vi "Modules - Station.vi"(8 "error in":errorcluster) -> (0 "error out":errorcluster)   [LabVIEW 2019]
uses:
  Controls/Station - Tab Test Type.ctl
  Controls/Station - Test Type.ctl
  Controls/Station-state.ctl
  Controls/Station - Data Structure.ctl
  Controls/eFGV States.ctl
  <vilib>/Utility/miscctls.llb/LVRowAndColumnTypeDef.ctl
  Controls/Global - Channel.vi
  Controls/Global - Unit.vi
  Controls/Global - Device.vi
  Controls/Global - Rendezvous.vi
panel:
  out "ID":string
  in  "Refresh Button":bool
  out "Main Tab":enum32{"Blank", "Edit"}(tab)
  out "Sub Tab":T1
  out "Unit PPT Triaxial Shear":string caption="Cell Pressure Transducer"
  out "Unit Disp Triaxial Shear":string caption="Cell Pressure Transducer"
  out "Unit LT Triaxial Shear":string caption="Cell Pressure Transducer"
  out "Unit VC Triaxial Shear":string caption="Cell Pressure Transducer"
  out "Unit BPT Triaxial Shear":string caption="Cell Pressure Transducer"
  out "Unit CPT Triaxial Shear":string caption="Cell Pressure Transducer"
  in  "VLC Triaxial Shear":u16(ring) caption="Vertical Load Control" items=["Please Select"]
  in  "BPC Triaxial Shear":u16(ring) caption="Back Pressure Control" items=["Please Select"]
  out "Disp Triaxial Shear":sgl caption="Dispalcement" format="%.5f"
  out "PPT Triaxial Shear":sgl caption="Pore Pressure Transduser" format="%.5f"
  out "LT Triaxial Shear":sgl caption="Load Tranduser" format="%.5f"
  out "BPT Triaxial Shear":sgl caption="Back Pressure Transducer" format="%.5f"
  out "VC Triaxial Shear":sgl caption="Volume Change" format="%.5f"
  out "CPT Triaxial Shear":sgl caption="Cell Pressure Transducer" format="%.5f"
  in  "CPC Triaxial Shear":u16(ring) caption="Cell Pressure Control" items=["Please Select"]
  in  "VLC Triaxial UU":u16(ring) caption="Vertical Load Control" items=["Please Select"]
  out "CPT Triaxial UU":sgl caption="Cell Pressure" format="%.5f"
  out "VLT Triaxial UU":sgl caption="Vertical Load" format="%.5f"
  out "PPT Triaxial UU":sgl caption="Pore Pressure" format="%.5f"
  out "Disp Triaxial UU":sgl caption="Displacement" format="%.5f"
  in  "CPC Triaxial UU":u16(ring) caption="Cell Pressure Control" items=["Please Select"]
  out "Unit CPT Triaxial UU":string caption="Cell Pressure Transducer"
  out "Unit VLT Triaxial UU":string caption="Cell Pressure Transducer"
  out "Unit Disp Triaxial UU":string caption="Cell Pressure Transducer"
  out "Unit PPT Triaxial UU":string caption="Cell Pressure Transducer"
  in  "HLC Shearbox":u16(ring) caption="Horinzontal Load Control" items=["Please Select"]
  out "LT Shearbox":sgl caption="Vertical Load Tranducer" format="%.5f"
  out "Disp Shearbox":sgl caption="Vertical Dispalcement" format="%.5f"
  out "H Dis Shearbox":sgl caption="Horizontal Dispalcement" format="%.5f"
  out "HLT Shearbox":sgl caption="Horinzontal Load Tranducer" format="%.5f"
  in  "VLC Shearbox":u16(ring) caption="Vertical Load Control" items=["Please Select"]
  out "Unit LT Shearbox":string caption="Cell Pressure Transducer"
  out "Unit Disp Shearbox":string caption="Cell Pressure Transducer"
  out "Unit HLT Shearbox":string caption="Cell Pressure Transducer"
  out "Unit H Dis Shearbox":string caption="Cell Pressure Transducer"
  in  "BPC2 Permeability":u16(ring) caption="Back Pressure 2 Control" items=["Please Select"]
  in  "BPC Permeability":u16(ring) caption="Back Pressure Control" items=["Please Select"]
  out "BPT2 Permeability":sgl caption="Back Pressure 2" format="%.5f"
  out "PPT Permeability":sgl caption="Pore Pressure" format="%.5f"
  out "OVC Permeability":sgl caption="Outlet Volume Change" format="%.5f"
  out "BPT Permeability":sgl caption="Back Pressure" format="%.5f"
  out "IVC Permeability":sgl caption="Inlet Volume Change" format="%.5f"
  out "CPT Permeability":sgl caption="Cell Pressure" format="%.5f"
  in  "CPC Permeability":u16(ring) caption="Cell Pressure Control" items=["Please Select"]
  out "Unit CPT Permeability":string caption="Cell Pressure Transducer"
  out "Unit BPT Permeability":string caption="Cell Pressure Transducer"
  out "Unit IVC Permeability":string caption="Cell Pressure Transducer"
  out "Unit BPT2 Permeability":string caption="Cell Pressure Transducer"
  out "Unit OVC Permeability":string caption="Cell Pressure Transducer"
  out "Unit PPT Permeability":string caption="Cell Pressure Transducer"
  out "Disp Consolidation":sgl caption="Dispalcement"
  out "LT Consolidation":sgl caption="Load Tranducer"
  in  "VLC Consolidation":u16(ring) caption="Vertical Load  Control" items=["Please Select"]
  out "Unit LT Consolidation":string caption="Cell Pressure Transducer"
  out "Unit Disp Consolidation":string caption="Cell Pressure Transducer"
  out "CPT Saturation":sgl caption="Cell Pressure Transducer" format="%.5f"
  out "VC Saturation":sgl caption="Volume Change" format="%.5f"
  out "BPT Saturation":sgl caption="Back Pressure Transducer" format="%.5f"
  out "PPT Saturation":sgl caption="Pore pressure Tranduser" format="%.5f"
  in  "CPC Saturation":u16(ring) caption="Cell Pressure Control" items=["Please Select"]
  in  "BPC Saturation":u16(ring) caption="Back Pressure Control" items=["Please Select"]
  out "Unit CPT Saturation":string caption="Cell Pressure Transducer"
  out "Unit BPT Saturation":string caption="Cell Pressure Transducer"
  out "Unit VC Saturation":string caption="Cell Pressure Transducer"
  out "Unit PPT Saturation":string caption="Cell Pressure Transducer"
  out "HD User Defined":sgl caption="Horizontal Displacement"
  out "HL User Defined":sgl caption="Horizontal Load"
  out "VD User Defined":sgl caption="Vertical Displacement"
  out "VC2 User Defined":sgl caption="Volume Change 2"
  out "VC1 User Defined":sgl caption="Volume Change 1"
  out "VL User Defined":sgl caption="Vertical Load"
  out "BPT2 User Defined":sgl caption="Back Pressure 2"
  out "PWP User Defined":sgl caption="Pore Water Pressure"
  out "BPT User Defined":sgl caption="Back Pressure"
  out "CPT User Defined":sgl caption="Cell Pressure"
  in  "HLC User Defined":u16(ring) caption="Horizontal Load Control" items=["Please Select"]
  in  "VLC User Defined":u16(ring) caption="Vertical Load Control" items=["Please Select"]
  in  "BPC2 User Defined":u16(ring) caption="Back Pressure 2 Control" items=["Please Select"]
  in  "BPC User Defined":u16(ring) caption="Back Pressure Control" items=["Please Select"]
  in  "CPC User Defined":u16(ring) caption="Cell Pressure Control" items=["Please Select"]
  out "Unit CPT User Defined":string caption="Cell Pressure Transducer"
  out "Unit BPT User Defined":string caption="Cell Pressure Transducer"
  out "Unit VC1 User Defined":string caption="Cell Pressure Transducer"
  out "Unit PWP User Defined":string caption="Cell Pressure Transducer"
  out "Unit BPT2 User Defined":string caption="Cell Pressure Transducer"
  out "Unit VC2 User Defined":string caption="Cell Pressure Transducer"
  out "Unit HD User Defined":string caption="Cell Pressure Transducer"
  out "Unit HL User Defined":string caption="Cell Pressure Transducer"
  out "Unit VD User Defined":string caption="Cell Pressure Transducer"
  out "Unit VL User Defined":string caption="Cell Pressure Transducer"
  in  "Test Type":T2 items=["Please Select", "Triaxial Shear", "Triaxial UU", "Shearbox", "Permeability", "Consolidation (Stepped Loading)/Swelling", "Saturation (Incremental)", "User Defined", "UCT", "Isotropic Consolidation", "Swelling Pressure"]
  in  "Station Name":string
  in  "save edit":bool
  in  "DELETE STATION":bool
  in  "Table":i32(listbox)
  in  "OK":bool
  in  "CREATE NEW STATION":bool
  # "*Double-Click to Edit / Delete"
  # "Live Reading"
  # "Live Reading"
  # "Live Reading"
  # "Live Reading"
  # "Live Reading"
  # "Live Reading"
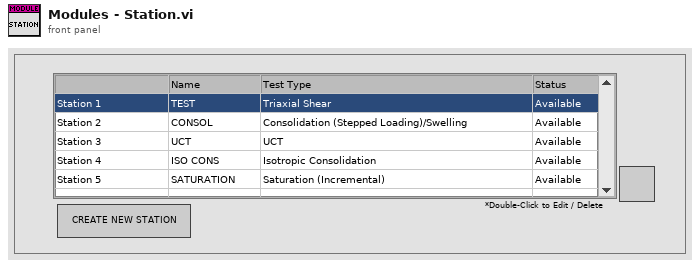
[diagram p1: front panel]
types:
  T1 = typedef "Station - Tab Test Type.ctl" = enum32{"Please Select", "Triaxial Shear", "Triaxial UU", "Shearbox", "Permeability", "Consolidation", "Saturation", "User Defined", "UCT", "Isotropic Consolidation"}
  T2 = typedef "Station - Test Type.ctl" = u16
  T3 = typedef "Station-state.ctl" = enum16{"Init", "Read Config", "Idle", "Delete", "Upload", "save edit", "update stationid", "Close", "Read sensor", "Exit"}
  T4 = enum32{"Please Select", "Triaxial Shear", "Triaxial UU", "Shearbox", "Permeability", "Consolidation", "Saturation", "User Defined"}
  T5 = typedef "Station - Data Structure.ctl" = cluster{"Table station":string[][], "Station Name":string, "EditRow":i32, "Station ID":string}
  T6 = enum32{"Invalid", "Standard", "Closed", "Hidden", "Minimized", "Maximized"}
  T7 = typedef "eFGV States.ctl" = enum16{"Init", "Read", "Write", "Exit"}
  T8 = typedef "Rendezvous RefNum" = refnum<k1>
  T9 = cluster{"Station Name":string, "Key Value":string[], "Key Names":string[]}[]
  T10 = typedef "UDP - Event.ctl" = u16
  T11 = typedef "UDP - Status.ctl" = u16
  T12 = cluster{"Channels":cluster{"Ch1":sgl, "Ch2":sgl, "Ch3":sgl, "Ch4":sgl, "Ch5":sgl, "Ch6":sgl, "Ch7":sgl, "Ch8":sgl, "Ch9":sgl, "Ch10":sgl, "Ch11":sgl, "Ch12":sgl, "Ch13":sgl, "Ch14":sgl, "Ch15":sgl, "Ch16":sgl}, "Event":T10, "Status":T11, "IP":string}[]
  T13 = cluster{"Name":string[], "Unit":string[], "Decimal Point":u8[], "Ch Log":u8[], "H Alarm":u8[], "L Alarm":u8[], "H Limit":sgl[], "L Limit":sgl[], "Filter":u8[], "Gain":u8[], "Calib Type":u32[]}[]
  T14 = cluster{"Channels":cluster{"Ch1":sgl, "Ch2":sgl, "Ch3":sgl, "Ch4":sgl, "Ch5":sgl, "Ch6":sgl, "Ch7":sgl, "Ch8":sgl, "Ch9":sgl, "Ch10":sgl, "Ch11":sgl, "Ch12":sgl, "Ch13":sgl, "Ch14":sgl, "Ch15":sgl, "Ch16":sgl}, "Event":T10, "Status":T11, "IP":string}
  T15 = cluster{"Name":string[], "Unit":string[], "Decimal Point":u8[], "Ch Log":u8[], "H Alarm":u8[], "L Alarm":u8[], "H Limit":sgl[], "L Limit":sgl[], "Filter":u8[], "Gain":u8[], "Calib Type":u32[]}
  T16 = cluster{"Station Name":string, "Key Value":string[], "Key Names":string[]}
  T17 = typedef "LVRowAndColumnTypeDef.ctl" = cluster{"Row":i32, "Column":i32}
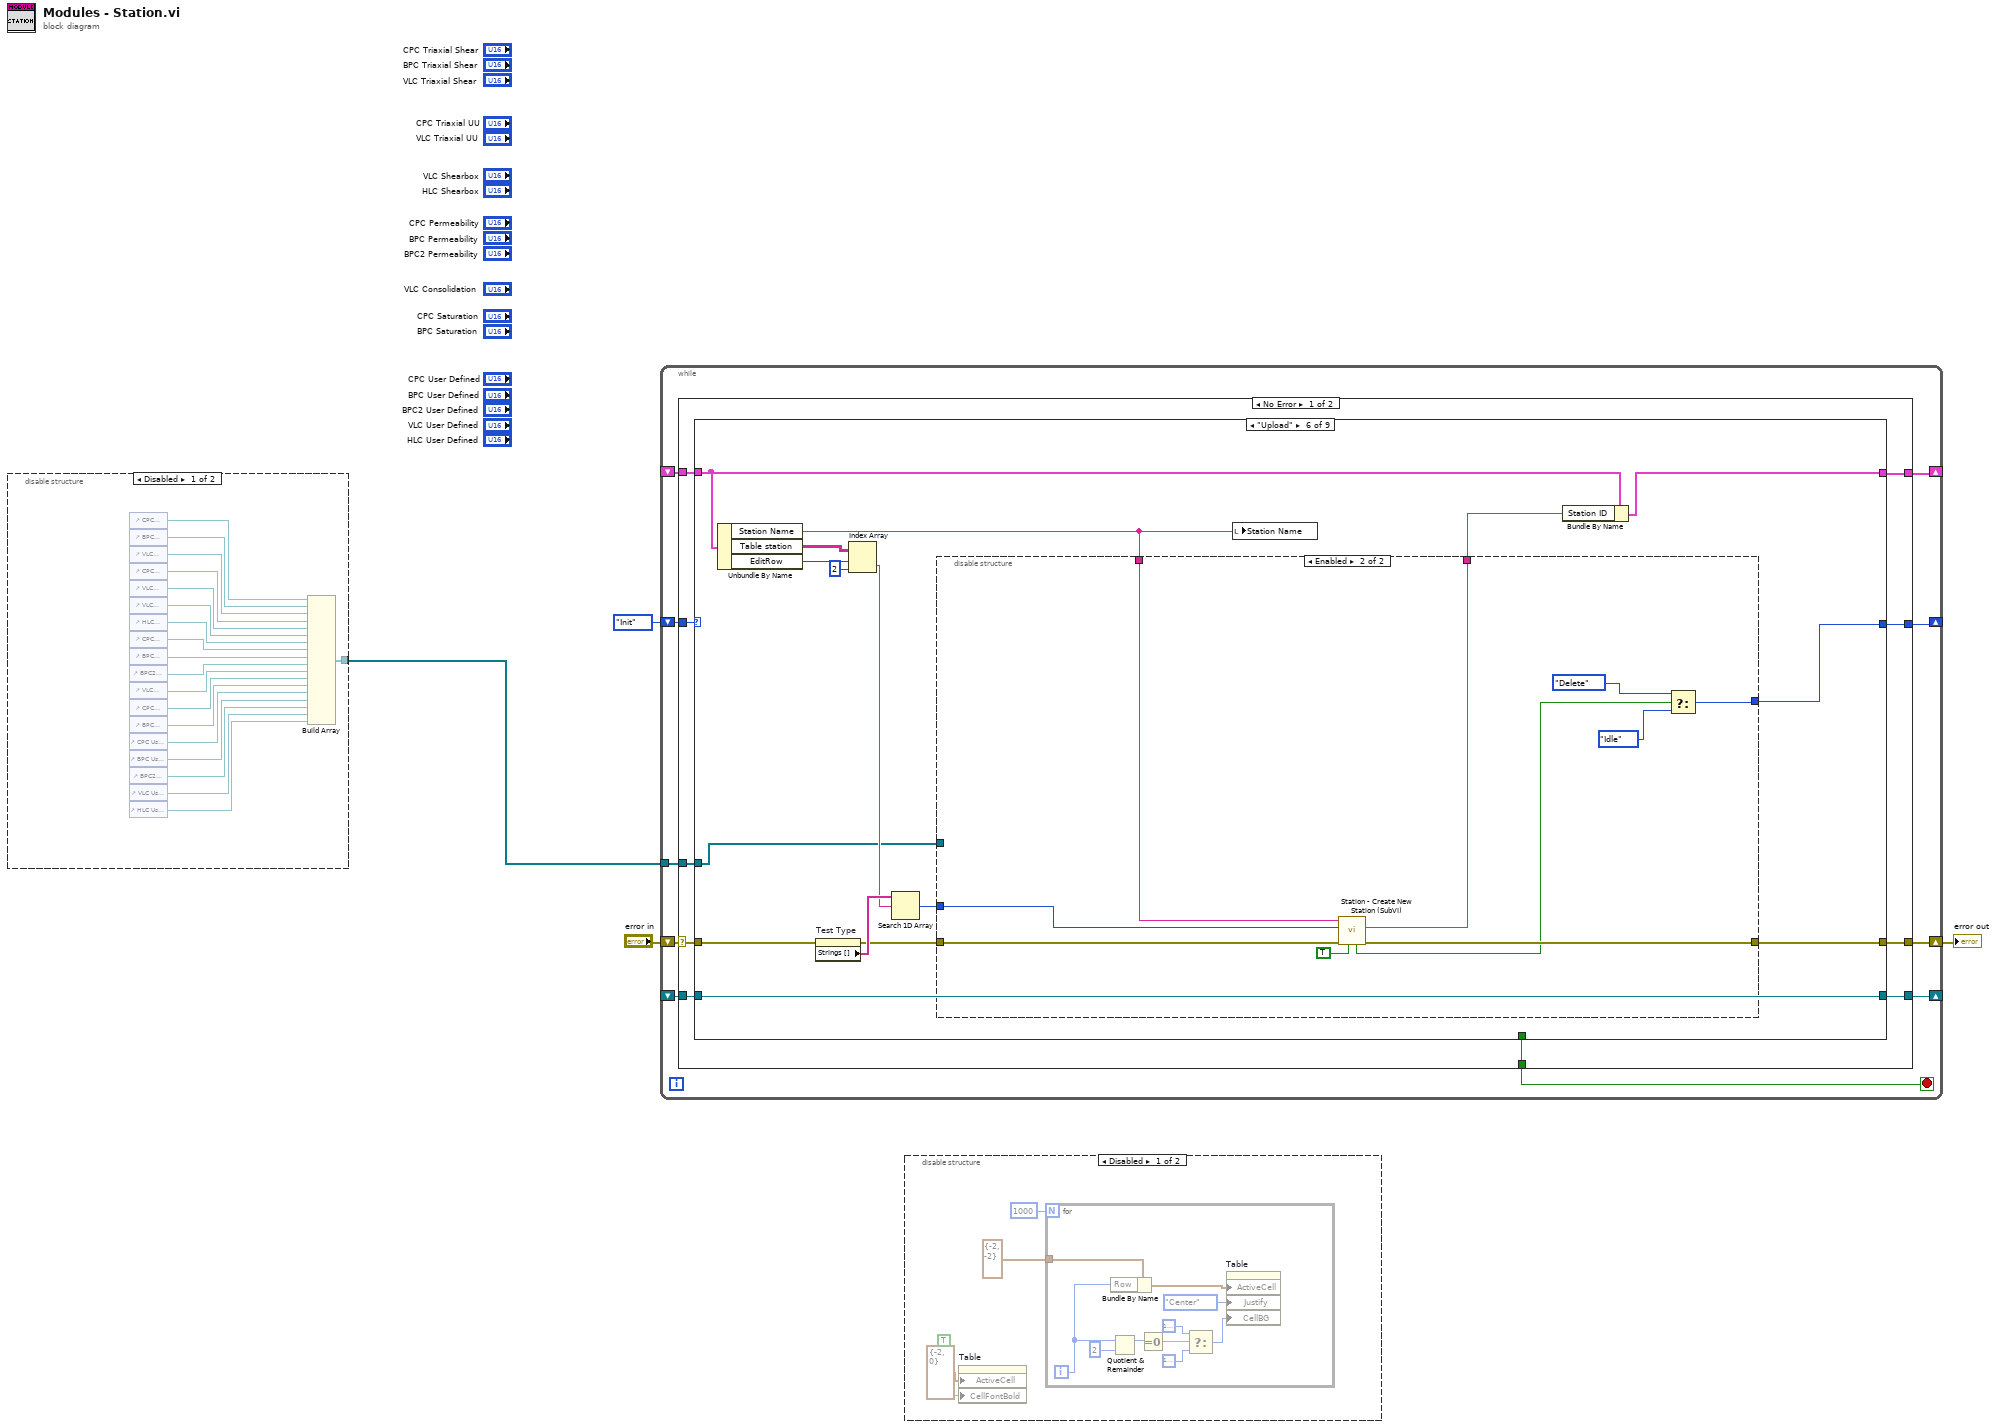
[diagram p0: block diagram]
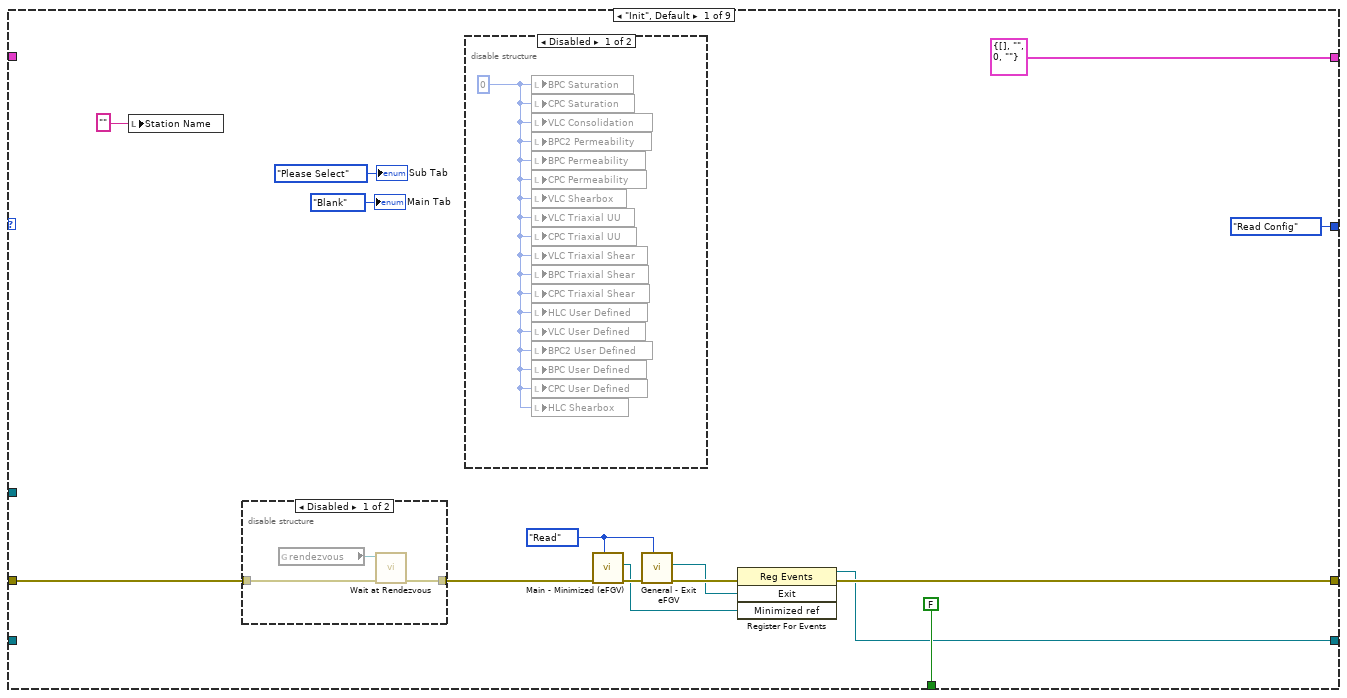
[diagram p3: hidden frame]
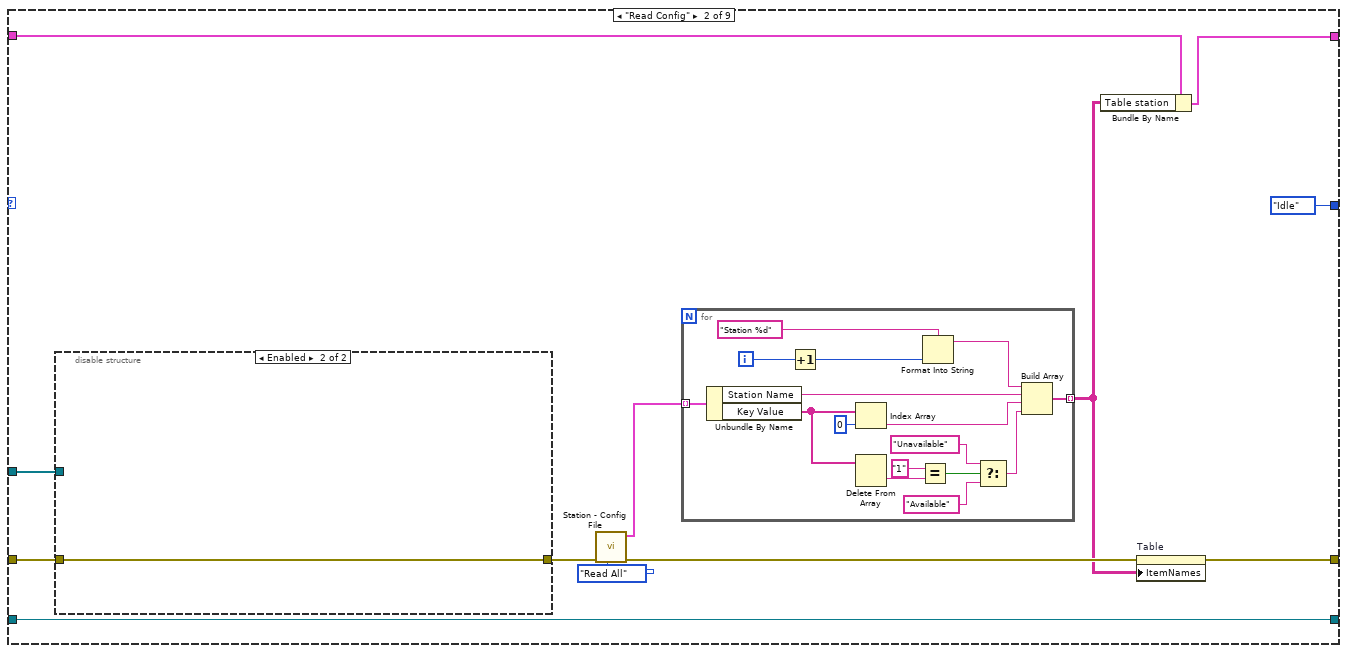
[diagram p6: hidden frame]
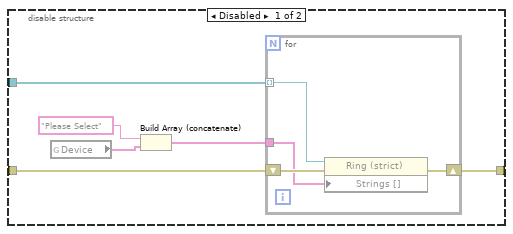
[diagram p7: hidden frame]
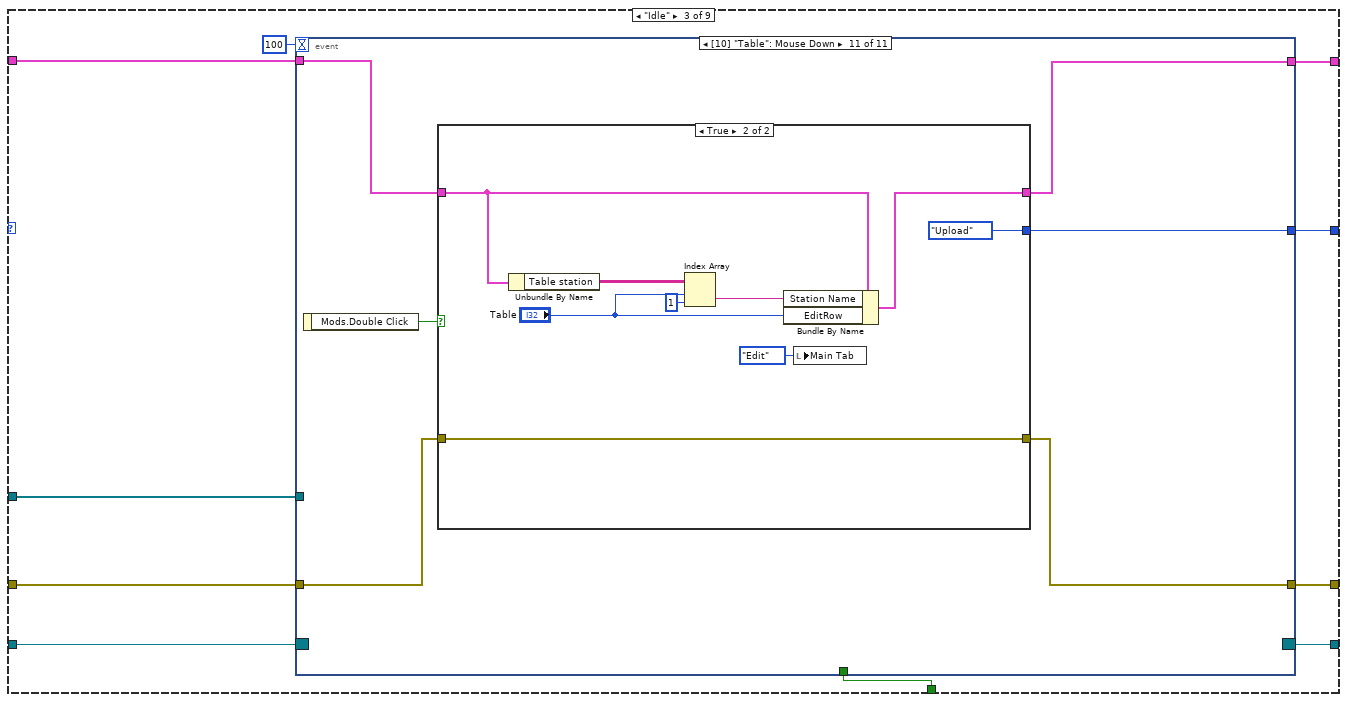
[diagram p8: hidden frame]
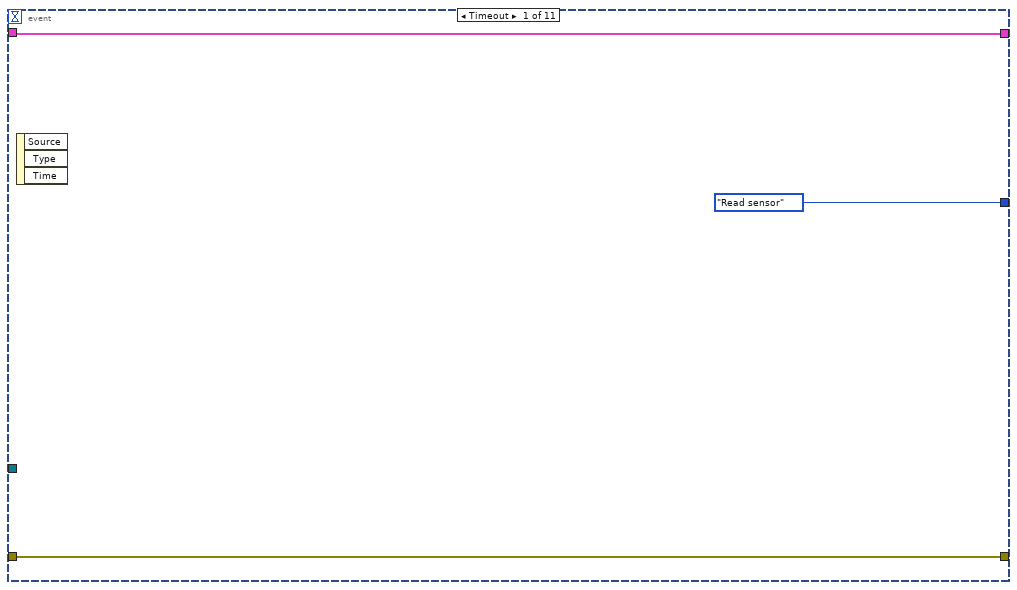
[diagram p9: hidden frame]
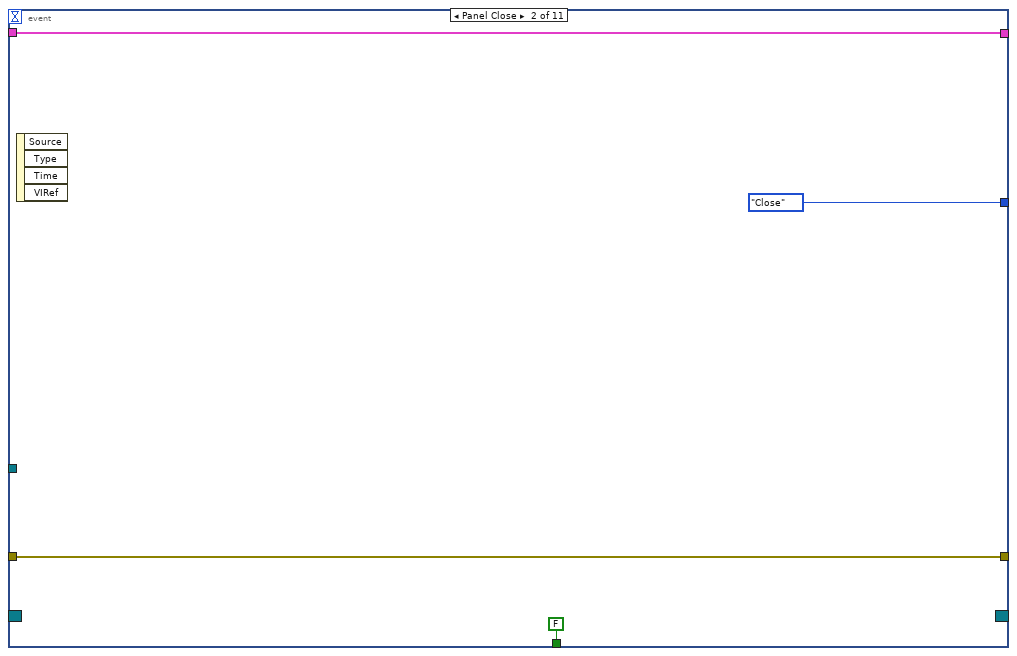
[diagram p10: hidden frame]
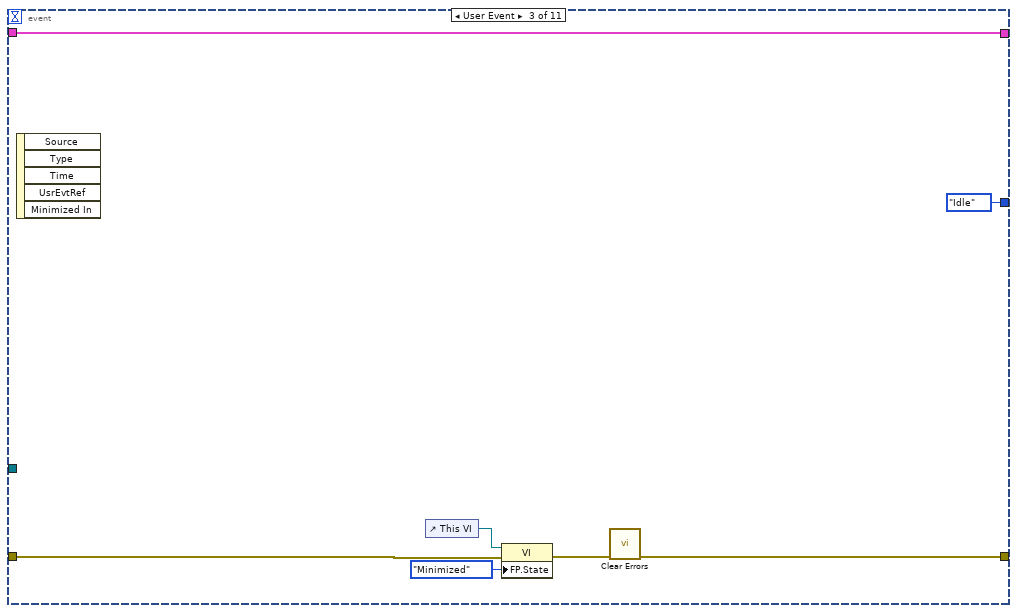
[diagram p11: hidden frame]
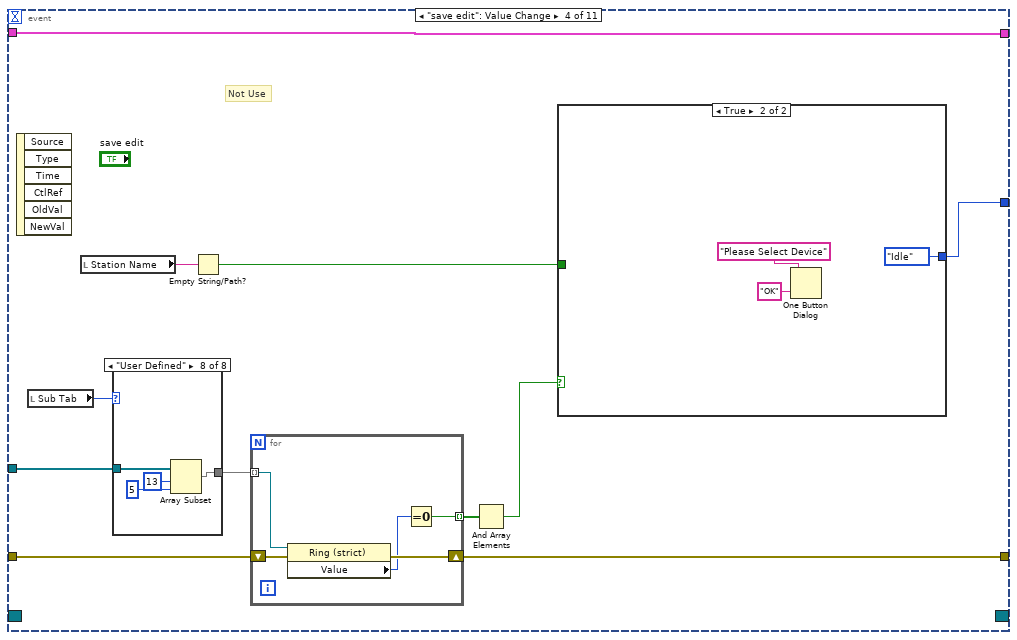
[diagram p12: hidden frame]
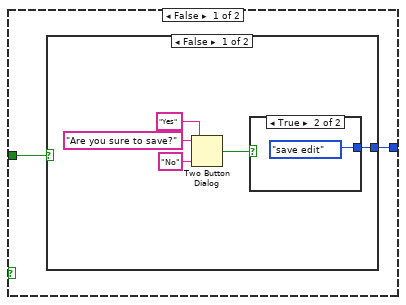
[diagram p13: hidden frame]
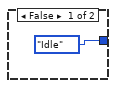
[diagram p14: hidden frame]
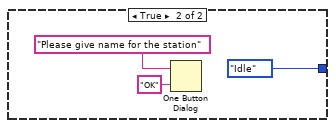
[diagram p15: hidden frame]
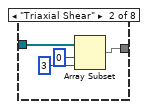
[diagram p17: hidden frame]
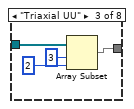
[diagram p18: hidden frame]
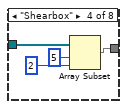
[diagram p19: hidden frame]
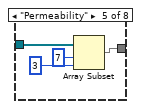
[diagram p20: hidden frame]
diagram:
  n1 = disable-structure shown="Disabled" {
    disable-tunnel: [w5 _] -> w1
    frame Disabled {
      n2 = control-ref of="CPC Triaxial Shear"() -> (w23:refnum<vi>)
      n3 = control-ref of="BPC Triaxial Shear"() -> (w22:refnum<vi>)
      n4 = control-ref of="VLC Triaxial Shear"() -> (w21:refnum<vi>)
      n5 = control-ref of="CPC Triaxial UU"() -> (w20:refnum<vi>)
      n6 = control-ref of="VLC Triaxial UU"() -> (w19:refnum<vi>)
      n7 = control-ref of="VLC Shearbox"() -> (w18:refnum<vi>)
      n8 = control-ref of="HLC Shearbox"() -> (w17:refnum<vi>)
      n9 = control-ref of="CPC Permeability"() -> (w16:refnum<vi>)
      n10 = control-ref of="BPC Permeability"() -> (w15:refnum<vi>)
      n11 = control-ref of="BPC2 Permeability"() -> (w14:refnum<vi>)
      n12 = control-ref of="VLC Consolidation"() -> (w13:refnum<vi>)
      n13 = control-ref of="CPC Saturation"() -> (w12:refnum<vi>)
      n14 = control-ref of="BPC Saturation"() -> (w11:refnum<vi>)
      n15 = control-ref of="CPC User Defined"() -> (w10:refnum<vi>)
      n16 = control-ref of="BPC User Defined"() -> (w9:refnum<vi>)
      n17 = control-ref of="BPC2 User Defined"() -> (w8:refnum<vi>)
      n18 = control-ref of="VLC User Defined"() -> (w7:refnum<vi>)
      n19 = control-ref of="HLC User Defined"() -> (w6:refnum<vi>)
      n20 = Build Array(w23, w22, w21, w20, w19, w18, w17, w16, w15, w14, w13, w12, w11, w10, w9, w8, w7, w6) -> (w5:refnum<vi>[])
    }
    frame Enabled {
    }
  }
  n21 = while {
    shift-right: [w32] -> w3
    shift-left: "error in" -> [w33]
    shift-right: [w30] -> _
    shift-left: Station-state."Init" -> [w31]
    shift-right: [w28] -> _
    shift-left: _ -> [w27]
    shift-right: [w26] -> _
    shift-left: _ -> [w25]
    tunnel: w1 -> [w24]
    stop <- w29 stop-if-true
    n22 = case shown="No Error" w33 {
      selector: w33 -> [w42 w711]
      tunnel: [w41 w712] -> w32
      tunnel: w31 -> [w43 _]
      tunnel: [w40 Station-state."Idle"] -> w30
      tunnel: [w39 _] -> w29
      tunnel: [w38 w721] -> w28
      tunnel: w27 -> [w37 w721]
      tunnel: [w36 w719] -> w26
      tunnel: w25 -> [w35 w719]
      tunnel: w24 -> [w34 _]
      frame No Error {
        n23 = case shown="\"Upload\"" w43 {
          tunnel: w42 -> [w48 w67 w111 w245 w528 w546 w629 w702 w704]
          tunnel: [w54 w64 w110 w244 w529 w541 w628 w696 w703] -> w41
          tunnel: [Station-state."Read Config" Station-state."Idle" w108 Station-state."Idle" Station-state."Read Config" w535 Station-state."Read Config" Station-state."Idle" Station-state."Exit"] -> w40
          tunnel: [FALSE _ w109 _ _ _ _ _ TRUE] -> w39
          tunnel: [T5 {"Table station"=[], "Station Name"="", "EditRow"=0, "Station ID"=""} w69 w106 w248 w533 w538 w626 w701 w710] -> w38
          tunnel: w37 -> [_ w70 w107 w248 w533 w537 w626 w701 w710]
          tunnel: [w52 w73 w104 w247 w532 w550 w630 w697 w709] -> w36
          tunnel: w35 -> [_ w73 w105 w247 w532 w550 w630 w697 w709]
          tunnel: w34 -> [_ w66 w102 w243 _ w539 w627 _ _]
          frame "Init", Default {
            w45 = eFGV_States."Read" ("eFGV States")
            n24 = local write "Station Name"("" ("New station name:")) -> ()
            n25 = disable-structure shown="Disabled" {
              disable-tunnel: [w62 _] -> w47
              disable-tunnel: w48 -> [w61 _]
              frame Disabled {
                n26 = global read "Global - Rendezvous.vi" "rendezvous"() -> (w60:T8)
                n27 = call <vilib>:"Wait at Rendezvous.vi"("error in (no error)"=w61, "rendezvous"=w60) -> ("error out"=w62:errorcluster)  [unwired: 3 in, 2 out]
              }
              frame Enabled {
              }
            }
            n28 = disable-structure shown="Disabled" {
              frame Disabled {
                w59 = 0
                n29 = local write "BPC Saturation"(w59) -> ()
                n30 = local write "CPC Saturation"(w59) -> ()
                n31 = local write "VLC Consolidation"(w59) -> ()
                n32 = local write "BPC2 Permeability"(w59) -> ()
                n33 = local write "BPC Permeability"(w59) -> ()
                n34 = local write "CPC Permeability"(w59) -> ()
                n35 = local write "VLC Shearbox"(w59) -> ()
                n36 = local write "VLC Triaxial UU"(w59) -> ()
                n37 = local write "CPC Triaxial UU"(w59) -> ()
                n38 = local write "VLC Triaxial Shear"(w59) -> ()
                n39 = local write "BPC Triaxial Shear"(w59) -> ()
                n40 = local write "CPC Triaxial Shear"(w59) -> ()
                n41 = local write "HLC User Defined"(w59) -> ()
                n42 = local write "VLC User Defined"(w59) -> ()
                n43 = local write "BPC2 User Defined"(w59) -> ()
                n44 = local write "BPC User Defined"(w59) -> ()
                n45 = local write "CPC User Defined"(w59) -> ()
                n46 = local write "HLC Shearbox"(w59) -> ()
              }
              frame Enabled {
              }
            }
            n47 = call "Main - Minimized (eFGV).vi"("Action"=w45, "error in"=w47) -> ("error out"=w46:errorcluster, "Minimized ref"=w44:refnum<user-event>)  [unwired: 7 in, 1 out]
            n48 = call "General - Exit eFGV.vi"("eFGV States"=w45, "error in (no error)"=w46) -> ("error out"=w55:errorcluster, "Exit"=w53:refnum<user-event>)  [unwired: 7 in, 1 out]
            n49 = register-events(error in=w55, w53, w44) -> (reference out=w52:refnum<event-registration>, error out=w54:errorcluster)  [unwired: 1 in]
            "Sub Tab" <- T4."Please Select" ("Sub Tab")
            "Main Tab" <- enum32{"Blank", "Edit"}."Blank" ("Main Tab")
          }
          frame "Read Config" {
            n50 = disable-structure shown="Enabled" {
              disable-tunnel: [w78 w85] -> w68
              disable-tunnel: w67 -> [w77 w85]
              disable-tunnel: w66 -> [w76 _]
              frame Disabled {
                n51 = global read "Global - Device.vi" "Device"() -> (w75:string[])
                n52 = Build Array (concatenate)("Please Select", w75) -> (w79:string[])
                n53 = for {
                  shift-right: [w83] -> w78
                  shift-left: w77 -> [w84]
                  tunnel: w76 -> [w82] mode=indexing
                  tunnel: w79 -> [w81]
                  n54 = property class="Ring (strict)"(reference=w82, error in=w84, "Strings []"=w81) -> (error out=w83:errorcluster)  [unwired: 1 out]
                }
              }
              frame Enabled {
              }
            }
            n55 = call "Station - Config File.vi"("Action"=enum16{"Write", "Read", "Read All", "Remove"}."Read All", "error in (no error)"=w68) -> ("error out"=w65:errorcluster, "Value Out"=w71:T9)  [unwired: 8 in]
            n56 = for {
              tunnel: w71 -> [w101] mode=indexing
              tunnel: [w95] -> w63 mode=indexing
              i -> [w87]
              n57 = Unbundle By Name(w101) -> ("Station Name"=w97:string, "Key Value"=w88:string[])
              n58 = Increment(x=w87) -> (x+1=w86:i32)
              n59 = Index Array(array=w88, index=0) -> (element=w96:string)
              n60 = Delete From Array(array=w88) -> (deleted portion=w94:string)  [unwired: 2 in, 1 out]
              n61 = Equal?(x="1", y=w94) -> (x = y?=w92:bool)
              n62 = Format Into String(format string="Station %d", w86) -> (resulting string=w98:string)  [unwired: 2 in, 1 out]
              n63 = Select(t="Unavailable" ("x"), s=w92, f="Available" ("x")) -> (s? t:f=w90:string)
              n64 = Build Array(w98, w97, w96, w90) -> (w95:string[])
            }
            n65 = Bundle By Name(cluster=w70, "Table station"=w63) -> (w69:T5)
            n66 = property on="Table" class="MCListbox (strict)"(error in=w65, "ItemNames"=w63) -> (error out=w64:errorcluster)  [unwired: 1 in, 1 out]
          }
          frame "Idle" {
            n67 = event shown="[10] \"Table\": Mouse Down" {
              selector: w105 -> [_ _ _ _ _ _ _ _ _ _ _]
              dyn-events: [_ _ _ _ _ _ _ _ _ _ _] -> w104
              timeout: 100 -> [_ _ _ _ _ _ _ _ _ _ _]
              tunnel: w111 -> [w112 w118 w120 w129 w186 w206 w209 w216 w220 w223 w225]
              tunnel: [w112 w118 w119 w126 w186 w206 w209 w215 w220 w223 w226] -> w110
              tunnel: [_ FALSE _ _ _ _ _ _ _ FALSE _] -> w109
              tunnel: [Station-state."Read sensor" Station-state."Close" Station-state."Idle" w134 Station-state."Idle" w202 Station-state."Read Config" w212 Station-state."Exit" Station-state."Close" w230] -> w108
              tunnel: w107 -> [w114 w117 w125 w136 w188 w198 w208 w217 w219 w222 w227]
              tunnel: [w114 w117 w125 w136 w188 w198 w208 w217 w219 w222 w228] -> w106
              tunnel: w102 -> [_ _ _ w132 _ _ _ _ _ _ _]
              event Timeout {
                n68 = event-data() -> ()  [unwired: 1 in, 3 out]
              }
              event Panel Close {
                n69 = event-data() -> ()  [unwired: 1 in, 4 out]
              }
              event User Event {
                n70 = event-data() -> ()  [unwired: 1 in, 5 out]
                n71 = control-ref of="This VI"() -> (w123:refnum<vi>)
                n72 = property class="VI"(reference=w123, error in=w120, "FP.State"=T6."Minimized" ("Front Panel Window:State")) -> (error out=w121:errorcluster)  [unwired: 1 out]
                n73 = call <vilib>:"Clear Errors.vi"("error in (no error)"=w121) -> ("error out"=w119:errorcluster)  [unwired: 5 in, 1 out]
              }
              event "save edit": Value Change {
                # "Not Use"
                n74 = event-data() -> ()  [unwired: 1 in, 6 out]
                n75 = local read "Sub Tab"() -> (w131:T1)
                n76 = local read "Station Name"() -> (w133:string)
                n77 = case shown="\"User Defined\"" w131 {
                  tunnel: w132 -> [_ w160 w162 w166 w170 w174 w178 w182]
                  tunnel: [_ w157 w161 w165 w169 w173 w177 w181] -> w130
                  frame "Please Select", Default {
                  }
                  frame "Triaxial Shear" {
                    n78 = Array Subset(array=w160, index=0, length=3) -> (w157:refnum<vi>[])
                  }
                  frame "Triaxial UU" {
                    n79 = Array Subset(array=w162, index=3, length=2) -> (w161:refnum<vi>[])
                  }
                  frame "Shearbox" {
                    n80 = Array Subset(array=w166, index=5, length=2) -> (w165:refnum<vi>[])
                  }
                  frame "Permeability" {
                    n81 = Array Subset(array=w170, index=7, length=3) -> (w169:refnum<vi>[])
                  }
                  frame "Consolidation" {
                    n82 = Array Subset(array=w174, index=10, length=1) -> (w173:refnum<vi>[])
                  }
                  frame "Saturation" {
                    n83 = Array Subset(array=w178, index=11, length=2) -> (w177:refnum<vi>[])
                  }
                  frame "User Defined" {
                    n84 = Array Subset(array=w182, index=13, length=5) -> (w181:refnum<vi>[])
                  }
                }
                n85 = Empty String/Path?(string/path=w133) -> (empty?=w135:bool)
                n86 = for {
                  tunnel: w130 -> [w154] mode=indexing
                  shift-right: [w155] -> w126
                  shift-left: w129 -> [w156]
                  tunnel: [w152] -> w128 mode=indexing
                  n87 = property class="Ring (strict)"(reference=w154, error in=w156) -> (error out=w155:errorcluster, "Value"=w153:u16)  [unwired: 1 out]
                  n88 = Equal To 0?(x=w153) -> (x = 0?=w152:bool)
                }
                n89 = And Array Elements(Boolean array=w128) -> (logical AND=w127:bool)
                n90 = case shown="True" w127 {
                  tunnel: w135 -> [w138 _]
                  tunnel: [w137 Station-state."Idle"] -> w134
                  frame False {
                    n91 = case shown="False" w138 {
                      tunnel: [w139 Station-state."Idle"] -> w137
                      frame False {
                        n92 = Two Button Dialog(message="Are you sure to save?", 1:"No" ("F button name (\"Cancel\")"), 2:"Yes" ("T button name (\"OK\")")) -> (T button?=w143:bool)
                        n93 = case shown="True" w143 {
                          tunnel: [Station-state."Idle" Station-state."save edit"] -> w139
                          frame False {
                          }
                          frame True {
                          }
                        }
                      }
                      frame True {
                        n94 = One Button Dialog(message="Please give name for the station", button name ("OK")="OK") -> ()  [unwired: 1 out]
                      }
                    }
                  }
                  frame True {
                    n95 = One Button Dialog(message="Please Select Device", button name ("OK")="OK") -> ()  [unwired: 1 out]
                  }
                }
              }
              event Value Change {
                # "Not Use"
                n96 = event-data() -> ("NewVal"=w187:T2)  [unwired: 1 in, 5 out]
                n97 = case shown="6" w187 {
                  tunnel: [Station_-_Tab_Test_Type."Please Select" ("Sub Tab") Station_-_Tab_Test_Type."Triaxial Shear" ("Sub Tab") Station_-_Tab_Test_Type."Triaxial UU" ("Sub Tab") Station_-_Tab_Test_Type."Shearbox" ("Sub Tab") Station_-_Tab_Test_Type."Permeability" ("Sub Tab") Station_-_Tab_Test_Type."Consolidation" ("Sub Tab") Station_-_Tab_Test_Type."Saturation" ("Sub Tab") Station_-_Tab_Test_Type."User Defined" ("Sub Tab")] -> w185
                  frame 0, Default {
                  }
                  frame 1 {
                  }
                  frame 2 {
                  }
                  frame 3 {
                  }
                  frame 4 {
                  }
                  frame 5 {
                  }
                  frame 6 {
                  }
                  frame 7 {
                  }
                }
                n98 = local write "Sub Tab"(w185) -> ()
              }
              event "DELETE STATION": Value Change {
                # "Not Use"
                n99 = event-data() -> ()  [unwired: 1 in, 6 out]
                n100 = Two Button Dialog(message="Are you sure to delete?", 1:"No" ("F button name (\"Cancel\")"), 2:"Yes" ("T button name (\"OK\")")) -> (T button?=w199:bool)
                n101 = Select(t=Station-state."Delete", s=w199, f=Station-state."Idle") -> (s? t:f=w202:T3)
              }
              event "Refresh Button": Value Change {
                n102 = event-data() -> ()  [unwired: 1 in, 6 out]
              }
              event "CREATE NEW STATION": Value Change {
                n103 = event-data() -> ()  [unwired: 1 in, 6 out]
                n104 = call "Station - Create New Station (SubVI).vi"("Load?"=FALSE, "error constant"=w216) -> ("error out"=w215:errorcluster, "ForceClose"=w214:bool)  [unwired: 6 in, 2 out]
                n105 = Select(t=Station-state."Idle", s=w214, f=Station-state."Read Config") -> (s? t:f=w212:T3)
              }
              event User Event {
                n106 = event-data() -> ()  [unwired: 1 in, 5 out]
              }
              event "OK": Value Change {
                n107 = event-data() -> ()  [unwired: 1 in, 6 out]
              }
              event "Table": Mouse Down {
                n108 = event-data() -> ("Mods.Double Click"=w229:bool)  [unwired: 1 in]
                n109 = case shown="True" w229 {
                  tunnel: [Station-state."Idle" Station-state."Upload"] -> w230
                  tunnel: w227 -> [w233 w237]
                  tunnel: [w233 w241] -> w228
                  tunnel: w225 -> [w231 w240]
                  tunnel: [w231 w240] -> w226
                  frame False {
                  }
                  frame True {
                    n110 = Unbundle By Name(w237) -> ("Table station"=w239:string[][])
                    n111 = Index Array(array=w239, index (row)="Table", index (col)=1 ("disabled index (col)")) -> (element=w234:string)
                    n112 = Bundle By Name(cluster=w237, "Station Name"=w234, "EditRow"="Table") -> (w241:T5)
                    n113 = local write "Main Tab"(enum32{"Blank", "Edit"}."Edit" ("Main Tab")) -> ()
                  }
                }
              }
            }
          }
          frame "Read sensor" {
            n114 = disable-structure shown="Enabled" {
              disable-tunnel: w245 -> [w253 w526]
              disable-tunnel: [w252 w526] -> w244
              disable-tunnel: w243 -> [w250 _]
              frame Disabled {
                # "not used"
                n115 = local read "Sub Tab"() -> (w251:T1)
                n116 = call "Station - Search Serial Number by Device Name.vi"("error in (no error)"=w253, "Array in"=w250) -> ("error out"=w255:errorcluster, "Index"=w249:i32[])  [unwired: 6 in, 2 out]
                n117 = case shown="\"User Defined\"" w251 {
                  tunnel: w249 -> [_ w501 w503 w507 w511 w515 w519 w523]
                  tunnel: [i32[] [] w498 w502 w506 w510 w514 w518 w522] -> w254
                  frame "Please Select", Default {
                  }
                  frame "Triaxial Shear" {
                    n118 = Array Subset(array=w501, index=0, length=3) -> (w498:i32[])
                  }
                  frame "Triaxial UU" {
                    n119 = Array Subset(array=w503, index=3, length=2) -> (w502:i32[])
                  }
                  frame "Shearbox" {
                    n120 = Array Subset(array=w507, index=5, length=2) -> (w506:i32[])
                  }
                  frame "Permeability" {
                    n121 = Array Subset(array=w511, index=7, length=3) -> (w510:i32[])
                  }
                  frame "Consolidation" {
                    n122 = Array Subset(array=w515, index=10, length=1) -> (w514:i32[])
                  }
                  frame "Saturation" {
                    n123 = Array Subset(array=w519, index=11, length=2) -> (w518:i32[])
                  }
                  frame "User Defined" {
                    n124 = Array Subset(array=w523, index=13, length=5) -> (w522:i32[])
                  }
                }
                n125 = for {
                  shift-right: [w270] -> w252
                  shift-left: w255 -> [w263]
                  tunnel: w254 -> [w262] mode=indexing
                  tunnel: w251 -> [w268]
                  i -> [w269]
                  n126 = global read "Global - Channel.vi" "Data"() -> (w257:T12)
                  n127 = global read "Global - Unit.vi" "Unit"() -> (w256:T13)
                  n128 = Index Array(array=w257, index=w262) -> (element=w261:T14)
                  n129 = Index Array(array=w256, index=w262) -> (element=w260:T15)
                  n130 = Unbundle By Name(w260) -> ("Ch1 Unit"=w265:string, "Ch2 Unit"=w264:string, "Ch2 Decimal"=w259:u8, "Ch1 Decimal"=w258:u8)
                  n131 = Unbundle By Name(w261) -> ("Ch1 Data"=w267:sgl, "Ch2 Data"=w266:sgl)
                  n132 = case shown="\"User Defined\"" w268 {
                    tunnel: [w271 w280 w316 w343 w370 w406 w424 w451] -> w270
                    tunnel: w263 -> [w271 w279 w315 w342 w369 w405 w423 w450]
                    tunnel: w269 -> [_ w278 w314 w341 w368 w404 w422 w449]
                    tunnel: w267 -> [_ w277 w313 w340 w367 w403 w421 w448]
                    tunnel: w265 -> [_ w276 w311 w338 w365 w401 w419 w446]
                    tunnel: w264 -> [_ w275 w310 w337 w364 w400 w418 w445]
                    tunnel: w266 -> [_ w274 w312 w339 w366 w402 w420 w447]
                    tunnel: w259 -> [_ w273 w309 w336 w363 w398 w416 w443]
                    tunnel: w258 -> [_ w272 w308 w335 w362 w399 w417 w444]
                    frame "Please Select", Default {
                    }
                    frame "Triaxial Shear" {
                      n133 = case shown="2" w278 {
                        tunnel: [w284 w293 w302] -> w280
                        tunnel: w279 -> [w283 w292 w301]
                        tunnel: w277 -> [w289 w298 w305]
                        tunnel: w276 -> [w288 w297 w307]
                        tunnel: w275 -> [w287 w296 w306]
                        tunnel: w274 -> [w286 w295 w304]
                        tunnel: w273 -> [w281 w290 w300]
                        tunnel: w272 -> [w282 w291 w299]
                        frame 0, Default {
                          n134 = property on="CPT Triaxial Shear" class="DigNum (strict)"(error in=w283, "Precision"=w282) -> (error out=w285:errorcluster)  [unwired: 1 in, 1 out]
                          n135 = property on="PPT Triaxial Shear" class="DigNum (strict)"(error in=w285, "Precision"=w281) -> (error out=w284:errorcluster)  [unwired: 1 in, 1 out]
                          "CPT Triaxial Shear" <- w289
                          "PPT Triaxial Shear" <- w286
                          "Unit CPT Triaxial Shear" <- w288
                          "Unit PPT Triaxial Shear" <- w287
                        }
                        frame 1 {
                          n136 = property on="BPT Triaxial Shear" class="DigNum (strict)"(error in=w292, "Precision"=w291) -> (error out=w294:errorcluster)  [unwired: 1 in, 1 out]
                          n137 = property on="VC Triaxial Shear" class="DigNum (strict)"(error in=w294, "Precision"=w290) -> (error out=w293:errorcluster)  [unwired: 1 in, 1 out]
                          "VC Triaxial Shear" <- w295
                          "BPT Triaxial Shear" <- w298
                          "Unit BPT Triaxial Shear" <- w297
                          "Unit VC Triaxial Shear" <- w296
                        }
                        frame 2 {
                          n138 = property on="LT Triaxial Shear" class="DigNum (strict)"(error in=w301, "Precision"=w299) -> (error out=w303:errorcluster)  [unwired: 1 in, 1 out]
                          n139 = property on="Disp Triaxial Shear" class="DigNum (strict)"(error in=w303, "Precision"=w300) -> (error out=w302:errorcluster)  [unwired: 1 in, 1 out]
                          "LT Triaxial Shear" <- w305
                          "Disp Triaxial Shear" <- w304
                          "Unit LT Triaxial Shear" <- w307
                          "Unit Disp Triaxial Shear" <- w306
                        }
                      }
                    }
                    frame "Triaxial UU" {
                      n140 = case shown="1" w314 {
                        tunnel: [w321 w331] -> w316
                        tunnel: w315 -> [w320 w330]
                        tunnel: w313 -> [w325 w334]
                        tunnel: w312 -> [w324 w333]
                        tunnel: w311 -> [w323 w326]
                        tunnel: w310 -> [w317 w327]
                        tunnel: w309 -> [w319 w329]
                        tunnel: w308 -> [w318 w328]
                        frame 0, Default {
                          n141 = property on="CPT Triaxial UU" class="DigNum (strict)"(error in=w320, "Precision"=w318) -> (error out=w322:errorcluster)  [unwired: 1 in, 1 out]
                          n142 = property on="PPT Triaxial UU" class="DigNum (strict)"(error in=w322, "Precision"=w319) -> (error out=w321:errorcluster)  [unwired: 1 in, 1 out]
                          "PPT Triaxial UU" <- w324
                          "CPT Triaxial UU" <- w325
                          "Unit CPT Triaxial UU" <- w323
                          "Unit PPT Triaxial UU" <- w317
                        }
                        frame 1 {
                          n143 = property on="VLT Triaxial UU" class="DigNum (strict)"(error in=w330, "Precision"=w328) -> (error out=w332:errorcluster)  [unwired: 1 in, 1 out]
                          n144 = property on="Disp Triaxial UU" class="DigNum (strict)"(error in=w332, "Precision"=w329) -> (error out=w331:errorcluster)  [unwired: 1 in, 1 out]
                          "Disp Triaxial UU" <- w333
                          "VLT Triaxial UU" <- w334
                          "Unit Disp Triaxial UU" <- w327
                          "Unit VLT Triaxial UU" <- w326
                        }
                      }
                    }
                    frame "Shearbox" {
                      n145 = case shown="0, Default" w341 {
                        tunnel: [w347 w356] -> w343
                        tunnel: w342 -> [w346 w355]
                        tunnel: w340 -> [w352 w361]
                        tunnel: w339 -> [w351 w360]
                        tunnel: w338 -> [w350 w359]
                        tunnel: w337 -> [w349 w358]
                        tunnel: w336 -> [w345 w354]
                        tunnel: w335 -> [w344 w353]
                        frame 0, Default {
                          n146 = property on="LT Shearbox" class="DigNum (strict)"(error in=w346, "Precision"=w344) -> (error out=w348:errorcluster)  [unwired: 1 in, 1 out]
                          n147 = property on="Disp Shearbox" class="DigNum (strict)"(error in=w348, "Precision"=w345) -> (error out=w347:errorcluster)  [unwired: 1 in, 1 out]
                          "LT Shearbox" <- w352
                          "Disp Shearbox" <- w351
                          "Unit Disp Shearbox" <- w349
                          "Unit LT Shearbox" <- w350
                        }
                        frame 1 {
                          n148 = property on="HLT Shearbox" class="DigNum (strict)"(error in=w355, "Precision"=w353) -> (error out=w357:errorcluster)  [unwired: 1 in, 1 out]
                          n149 = property on="H Dis Shearbox" class="DigNum (strict)"(error in=w357, "Precision"=w354) -> (error out=w356:errorcluster)  [unwired: 1 in, 1 out]
                          "HLT Shearbox" <- w361
                          "H Dis Shearbox" <- w360
                          "Unit HLT Shearbox" <- w359
                          "Unit H Dis Shearbox" <- w358
                        }
                      }
                    }
                    frame "Permeability" {
                      n150 = case shown="0, Default" w368 {
                        tunnel: [w374 w383 w392] -> w370
                        tunnel: w369 -> [w373 w382 w391]
                        tunnel: w367 -> [w379 w388 w397]
                        tunnel: w366 -> [w378 w387 w396]
                        tunnel: w365 -> [w377 w386 w395]
                        tunnel: w364 -> [w376 w385 w394]
                        tunnel: w363 -> [w372 w381 w389]
                        tunnel: w362 -> [w371 w380 w390]
                        frame 0, Default {
                          n151 = property on="CPT Permeability" class="DigNum (strict)"(error in=w373, "Precision"=w371) -> (error out=w375:errorcluster)  [unwired: 1 in, 1 out]
                          n152 = property on="PPT Permeability" class="DigNum (strict)"(error in=w375, "Precision"=w372) -> (error out=w374:errorcluster)  [unwired: 1 in, 1 out]
                          "CPT Permeability" <- w379
                          "PPT Permeability" <- w378
                          "Unit CPT Permeability" <- w377
                          "Unit PPT Permeability" <- w376
                        }
                        frame 1 {
                          n153 = property on="BPT Permeability" class="DigNum (strict)"(error in=w382, "Precision"=w380) -> (error out=w384:errorcluster)  [unwired: 1 in, 1 out]
                          n154 = property on="IVC Permeability" class="DigNum (strict)"(error in=w384, "Precision"=w381) -> (error out=w383:errorcluster)  [unwired: 1 in, 1 out]
                          "IVC Permeability" <- w387
                          "BPT Permeability" <- w388
                          "Unit BPT Permeability" <- w386
                          "Unit IVC Permeability" <- w385
                        }
                        frame 2 {
                          n155 = property on="BPT2 Permeability" class="DigNum (strict)"(error in=w391, "Precision"=w390) -> (error out=w393:errorcluster)  [unwired: 1 in, 1 out]
                          n156 = property on="OVC Permeability" class="DigNum (strict)"(error in=w393, "Precision"=w389) -> (error out=w392:errorcluster)  [unwired: 1 in, 1 out]
                          "OVC Permeability" <- w396
                          "BPT2 Permeability" <- w397
                          "Unit BPT2 Permeability" <- w395
                          "Unit OVC Permeability" <- w394
                        }
                      }
                    }
                    frame "Consolidation" {
                      n157 = case shown="0, Default" w404 {
                        tunnel: [w410] -> w406
                        tunnel: w405 -> [w409]
                        tunnel: w403 -> [w415]
                        tunnel: w402 -> [w414]
                        tunnel: w401 -> [w413]
                        tunnel: w400 -> [w412]
                        tunnel: w399 -> [w408]
                        tunnel: w398 -> [w407]
                        frame 0, Default {
                          n158 = property on="LT Consolidation" class="DigNum (strict)"(error in=w409, "Precision"=w408) -> (error out=w411:errorcluster)  [unwired: 1 in, 1 out]
                          n159 = property on="Disp Consolidation" class="DigNum (strict)"(error in=w411, "Precision"=w407) -> (error out=w410:errorcluster)  [unwired: 1 in, 1 out]
                          "LT Consolidation" <- w415
                          "Disp Consolidation" <- w414
                          "Unit LT Consolidation" <- w413
                          "Unit Disp Consolidation" <- w412
                        }
                      }
                    }
                    frame "Saturation" {
                      n160 = case shown="0, Default" w422 {
                        tunnel: [w428 w437] -> w424
                        tunnel: w423 -> [w427 w436]
                        tunnel: w421 -> [w433 w442]
                        tunnel: w420 -> [w432 w441]
                        tunnel: w419 -> [w431 w440]
                        tunnel: w418 -> [w430 w439]
                        tunnel: w417 -> [w426 w435]
                        tunnel: w416 -> [w425 w434]
                        frame 0, Default {
                          n161 = property on="CPT Saturation" class="DigNum (strict)"(error in=w427, "Precision"=w426) -> (error out=w429:errorcluster)  [unwired: 1 in, 1 out]
                          n162 = property on="PPT Saturation" class="DigNum (strict)"(error in=w429, "Precision"=w425) -> (error out=w428:errorcluster)  [unwired: 1 in, 1 out]
                          "CPT Saturation" <- w433
                          "PPT Saturation" <- w432
                          "Unit CPT Saturation" <- w431
                          "Unit PPT Saturation" <- w430
                        }
                        frame 1 {
                          n163 = property on="BPT Saturation" class="DigNum (strict)"(error in=w436, "Precision"=w435) -> (error out=w438:errorcluster)  [unwired: 1 in, 1 out]
                          n164 = property on="VC Saturation" class="DigNum (strict)"(error in=w438, "Precision"=w434) -> (error out=w437:errorcluster)  [unwired: 1 in, 1 out]
                          "BPT Saturation" <- w442
                          "VC Saturation" <- w441
                          "Unit BPT Saturation" <- w440
                          "Unit VC Saturation" <- w439
                        }
                      }
                    }
                    frame "User Defined" {
                      n165 = case shown="0, Default" w449 {
                        tunnel: [w455 w464 w473 w482 w491] -> w451
                        tunnel: w450 -> [w454 w463 w472 w481 w490]
                        tunnel: w448 -> [w460 w469 w478 w487 w496]
                        tunnel: w447 -> [w459 w468 w477 w486 w495]
                        tunnel: w446 -> [w458 w467 w476 w485 w494]
                        tunnel: w445 -> [w457 w466 w475 w484 w493]
                        tunnel: w444 -> [w453 w462 w471 w479 w489]
                        tunnel: w443 -> [w452 w461 w470 w480 w488]
                        frame 0, Default {
                          n166 = property on="CPT User Defined" class="DigNum (strict)"(error in=w454, "Precision"=w453) -> (error out=w456:errorcluster)  [unwired: 1 in, 1 out]
                          n167 = property on="PWP User Defined" class="DigNum (strict)"(error in=w456, "Precision"=w452) -> (error out=w455:errorcluster)  [unwired: 1 in, 1 out]
                          "CPT User Defined" <- w460
                          "PWP User Defined" <- w459
                          "Unit CPT User Defined" <- w458
                          "Unit PWP User Defined" <- w457
                        }
                        frame 1 {
                          n168 = property on="BPT User Defined" class="DigNum (strict)"(error in=w463, "Precision"=w462) -> (error out=w465:errorcluster)  [unwired: 1 in, 1 out]
                          n169 = property on="VC1 User Defined" class="DigNum (strict)"(error in=w465, "Precision"=w461) -> (error out=w464:errorcluster)  [unwired: 1 in, 1 out]
                          "BPT User Defined" <- w469
                          "VC1 User Defined" <- w468
                          "Unit BPT User Defined" <- w467
                          "Unit VC1 User Defined" <- w466
                        }
                        frame 2 {
                          n170 = property on="BPT2 User Defined" class="DigNum (strict)"(error in=w472, "Precision"=w471) -> (error out=w474:errorcluster)  [unwired: 1 in, 1 out]
                          n171 = property on="VC2 User Defined" class="DigNum (strict)"(error in=w474, "Precision"=w470) -> (error out=w473:errorcluster)  [unwired: 1 in, 1 out]
                          "BPT2 User Defined" <- w478
                          "VC2 User Defined" <- w477
                          "Unit BPT2 User Defined" <- w476
                          "Unit VC2 User Defined" <- w475
                        }
                        frame 3 {
                          n172 = property on="VL User Defined" class="DigNum (strict)"(error in=w481, "Precision"=w479) -> (error out=w483:errorcluster)  [unwired: 1 in, 1 out]
                          n173 = property on="VD User Defined" class="DigNum (strict)"(error in=w483, "Precision"=w480) -> (error out=w482:errorcluster)  [unwired: 1 in, 1 out]
                          "VL User Defined" <- w487
                          "VD User Defined" <- w486
                          "Unit VD User Defined" <- w484
                          "Unit VL User Defined" <- w485
                        }
                        frame 4 {
                          n174 = property on="HL User Defined" class="DigNum (strict)"(error in=w490, "Precision"=w489) -> (error out=w492:errorcluster)  [unwired: 1 in, 1 out]
                          n175 = property on="HD User Defined" class="DigNum (strict)"(error in=w492, "Precision"=w488) -> (error out=w491:errorcluster)  [unwired: 1 in, 1 out]
                          "HD User Defined" <- w495
                          "HL User Defined" <- w496
                          "Unit HD User Defined" <- w493
                          "Unit HL User Defined" <- w494
                        }
                      }
                    }
                  }
                }
              }
              frame Enabled {
              }
            }
          }
          frame "Delete" {
            n176 = Unbundle By Name(w533) -> ("Station Name"=w527:string)
            n177 = call "Station - Config File.vi"("Action"=enum16{"Write", "Read", "Read All", "Remove"}."Remove", "error in (no error)"=w528, "Station Name"=w527) -> ("error out"=w529:errorcluster)  [unwired: 7 in, 1 out]
            n178 = local write "Main Tab"(enum32{"Blank", "Edit"}."Blank" ("Main Tab")) -> ()
          }
          frame "Upload" {
            n179 = Unbundle By Name(w537) -> ("Station Name"=w542:string, "Table station"=w549:string[][], "EditRow"=w548:i32)
            n180 = property on="Test Type" class="Ring (strict)"(error in=w546) -> (error out=w543:errorcluster, "Strings []"=w545:string[])  [unwired: 1 in, 1 out]
            n181 = Index Array(array=w549, index (row)=w548, index (col)=2 ("disabled index (col)")) -> (element=w544:string)
            n182 = Search 1D Array(1D array=w545, element=w544) -> (index of element=w540:i32)  [unwired: 1 in]
            n183 = disable-structure shown="Enabled" {
              disable-tunnel: w543 -> [w571 w624]
              disable-tunnel: w542 -> [w568 w621]
              disable-tunnel: [w559 w623] -> w541
              disable-tunnel: w540 -> [w558 w622]
              disable-tunnel: w539 -> [w556 _]
              disable-tunnel: [w551 w620] -> w536
              disable-tunnel: [_ w616] -> w535
              frame Disabled {
                n184 = case shown="7" w558 {
                  tunnel: [string[] [] string[] ["Test Type", "CPC Triaxial Shear", "BPC Triaxial Shear", "VLC Triaxial Shear", "Status"] string[] ["Test Type", "CPC Triaxial UU", "VLC Triaxial UU", "Status"] string[] ["Test Type", "VLC Shearbox", "HLC Shearbox", "Status"] string[] ["Test Type", "CPC Permeability", "BPC Permeability", "BPC2 Permeability", "Status"] string[] ["Test Type", "VLC Consolidation", "Status"] string[] ["Test Type", "CPC Saturation", "BPC Saturation", "Status"] string[] ["Test Type", "CPC User Defined", "BPC User Defined", "BPC2 User Defined", "VLC User Defined", "HLC User Defined", "Status"]] -> w557
                  tunnel: w556 -> [_ w577 w580 w585 w590 w595 w600 w605]
                  tunnel: [refnum<vi>[] [] w574 w579 w584 w589 w594 w599 w604] -> w555
                  frame 0, Default {
                  }
                  frame 1 {
                    n185 = Array Subset(array=w577, index=0, length=3) -> (w574:refnum<vi>[])
                  }
                  frame 2 {
                    n186 = Array Subset(array=w580, index=3, length=2) -> (w579:refnum<vi>[])
                  }
                  frame 3 {
                    n187 = Array Subset(array=w585, index=5, length=2) -> (w584:refnum<vi>[])
                  }
                  frame 4 {
                    n188 = Array Subset(array=w590, index=7, length=3) -> (w589:refnum<vi>[])
                  }
                  frame 5 {
                    n189 = Array Subset(array=w595, index=10, length=1) -> (w594:refnum<vi>[])
                  }
                  frame 6 {
                    n190 = Array Subset(array=w600, index=11, length=2) -> (w599:refnum<vi>[])
                  }
                  frame 7 {
                    n191 = Array Subset(array=w605, index=13, length=5) -> (w604:refnum<vi>[])
                  }
                }
                n192 = property on="Test Type" class="Ring (strict)"(error in=w571, "Val(Sgnl)"=w558) -> (error out=w569:errorcluster)  [unwired: 1 in, 1 out]
                n193 = call "Station - Config File.vi"("Action"=enum16{"Write", "Read", "Read All", "Remove"}."Read", "error in (no error)"=w569, "Key Name"=w557, "Station Name"=w568) -> ("error out"=w560:errorcluster, "Value Out"=w567:T9)  [unwired: 6 in]
                n194 = Index Array(array=w567) -> (element=w566:T16)  [unwired: 1 in]
                n195 = Unbundle By Name(w566) -> ("Key Value"=w565:string[])
                n196 = Delete From Array(array=w565) -> (array with subset deleted=w564:string[])  [unwired: 2 in, 1 out]
                n197 = Delete From Array(array=w564, length=2, index=0) -> (deleted portion=w553:string[], array with subset deleted=w561:string[])
                n198 = global read "Global - Device.vi" "Device"() -> (w554:string[])
                n199 = Index Array(array=w553, index=1) -> (element=w551:string)
                "ID" <- w551
                n200 = for {
                  tunnel: w561 -> [w614] mode=indexing
                  tunnel: w554 -> [w615]
                  shift-right: [w612] -> w559
                  shift-left: w560 -> [w613]
                  tunnel: w555 -> [w611] mode=indexing
                  n201 = Search 1D Array(1D array=w615, element=w614) -> (index of element=w610:i32)  [unwired: 1 in]
                  n202 = Increment(x=w610) -> (x+1=w609:i32)
                  n203 = property class="Ring (strict)"(reference=w611, error in=w613, "Value"=w609) -> (error out=w612:errorcluster)  [unwired: 1 out]
                }
              }
              frame Enabled {
                n204 = call "Station - Create New Station (SubVI).vi"("Load?"=TRUE, "error constant"=w624, "Test Type"=w622, "Station Name"=w621) -> ("error out"=w623:errorcluster, "Station ID"=w620:string, "Delete?"=w617:bool)  [unwired: 4 in, 1 out]
                n205 = Select(t=Station-state."Delete", s=w617, f=Station-state."Idle") -> (s? t:f=w616:T3)
              }
            }
            n206 = local write "Station Name"(w542) -> ()
            n207 = Bundle By Name(cluster=w537, "Station ID"=w536) -> (w538:T5)
          }
          frame "save edit" {
            n208 = disable-structure shown="Disabled" {
              disable-tunnel: w629 -> [w643 w695]
              disable-tunnel: [w642 w695] -> w628
              disable-tunnel: w627 -> [w641 _]
              disable-tunnel: w626 -> [w633 _]
              frame Disabled {
                # "not use"
                n209 = for {
                  shift-right: [w656] -> w651
                  shift-left: w643 -> [w657]
                  tunnel: w641 -> [w655] mode=indexing
                  tunnel: [w654] -> w650 mode=indexing
                  n210 = property class="Ring (strict)"(reference=w655, error in=w657) -> (error out=w656:errorcluster, "RingText.Text"=w654:string)  [unwired: 1 out]
                }
                n211 = local read "Sub Tab"() -> (w640:T1)
                n212 = case shown="\"User Defined\"" w640 {
                  tunnel: [string[] [] string[] ["Test Type", "CPC Triaxial Shear", "BPC Triaxial Shear", "VLC Triaxial Shear", "Status"] string[] ["Test Type", "CPC Triaxial UU", "VLC Triaxial UU", "Status"] string[] ["Test Type", "VLC Shearbox", "HLC Shearbox", "Status"] string[] ["Test Type", "CPC Permeability", "BPC Permeability", "BPC2 Permeability", "Status"] string[] ["Test Type", "VLC Consolidation", "Status"] string[] ["Test Type", "CPC Saturation", "BPC Saturation", "Status"] string[] ["Test Type", "CPC User Defined", "BPC User Defined", "BPC2 User Defined", "VLC User Defined", "HLC User Defined", "Status"]] -> w636
                  tunnel: w650 -> [_ w663 w666 w671 w676 w681 w686 w691]
                  tunnel: [string[] [] w660 w665 w670 w675 w680 w685 w690] -> w649
                  frame "Please Select", Default {
                  }
                  frame "Triaxial Shear" {
                    n213 = Array Subset(array=w663, index=0, length=3) -> (w660:string[])
                  }
                  frame "Triaxial UU" {
                    n214 = Array Subset(array=w666, index=3, length=2) -> (w665:string[])
                  }
                  frame "Shearbox" {
                    n215 = Array Subset(array=w671, index=5, length=2) -> (w670:string[])
                  }
                  frame "Permeability" {
                    n216 = Array Subset(array=w676, index=7, length=3) -> (w675:string[])
                  }
                  frame "Consolidation" {
                    n217 = Array Subset(array=w681, index=10, length=1) -> (w680:string[])
                  }
                  frame "Saturation" {
                    n218 = Array Subset(array=w686, index=11, length=2) -> (w685:string[])
                  }
                  frame "User Defined" {
                    n219 = Array Subset(array=w691, index=13, length=5) -> (w690:string[])
                  }
                }
                n220 = Unbundle By Name(w633) -> ("Station ID"=w632:string)
                n221 = property on="Test Type" class="Ring (strict)"(error in=w651) -> (error out=w652:errorcluster, "RingText.Text"=w648:string)  [unwired: 1 in, 1 out]
                n222 = To Lower Case(string="Station Name") -> (all lower case string=w634:string)
                n223 = Insert Into Array(array=w649, index=0, new element #1=w648, new element #2=w632) -> (w645:string[])
                n224 = Build Array (concatenate)(w645, "0" ("String")) -> (w644:string[])
                n225 = Insert Into Array(array=w636, index=1, new element="ID" ("new element/subarray")) -> (w635:string[])
                n226 = call "Station - Config File.vi"("Action"=enum16{"Write", "Read", "Read All", "Remove"}."Write", "error in (no error)"=w652, "Value"=w644, "Key Name"=w635, "Station Name"=w634) -> ("error out"=w642:errorcluster)  [unwired: 5 in, 1 out]
              }
              frame Enabled {
              }
            }
          }
          frame "Close" {
            n227 = control-ref of="This VI"() -> (w698:refnum<vi>)
            n228 = invoke class="VI" method="FP.Close"(reference=w698, error in=w702) -> (error out=w699:errorcluster)  [unwired: 1 in, 2 out]
            n229 = call <vilib>:"Clear Errors.vi"("error in (no error)"=w699) -> ("error out"=w696:errorcluster)  [unwired: 5 in, 1 out]
          }
          frame "Exit" {
            n230 = control-ref of="This VI"() -> (w706:refnum<vi>)
            n231 = invoke class="VI" method="FP.Close"(reference=w706, error in=w704) -> (error out=w705:errorcluster)  [unwired: 1 in, 2 out]
            n232 = call <vilib>:"Clear Errors.vi"("error in (no error)"=w705) -> ("error out"=w703:errorcluster)  [unwired: 5 in, 1 out]
          }
        }
      }
      frame Error {
        n233 = Unbundle By Name(w711) -> ("source"=w716:string)
        n234 = call <vilib>:"Clear Errors.vi"("error in (no error)"=w711) -> ("error out"=w713:errorcluster)  [unwired: 5 in, 1 out]
        n235 = Concatenate Strings("Station" ("string"), " - " ("string"), w716) -> (w714:string)
        n236 = call "General - Error Log eFGV.vi"("eFGV States"=eFGV_States."Write", "error in (no error)"=w713, "Error In"=w714) -> ("error out"=w712:errorcluster)  [unwired: 6 in, 2 out]
        n237 = Wait (ms)(milliseconds to wait=u32 100) -> ()  [unwired: 1 out]
      }
    }
  }
  "error out" <- w3
  n238 = disable-structure shown="Disabled" {
    frame Disabled {
      n239 = property on="Table" class="MCListbox (strict)"("ActiveCell"=T17 {"Row"=-2, "Column"=0} ("Active Cell:Active Cell"), "CellFontBold"=TRUE ("Active Cell:Cell Font:Bold")) -> ()  [unwired: 2 in, 2 out]
      n240 = for {
        N: 1000 -> [_]
        tunnel: T17 {"Row"=-2, "Column"=-2} ("Active Cell:Active Cell") -> [w734]
        i -> [w730]
        n241 = Bundle By Name(cluster=w734, "Row"=w730) -> (w735:T17)
        n242 = Quotient & Remainder(x=w730, y=2) -> (x-y*floor(x/y)=w728:i32)  [unwired: 1 out]
        n243 = Equal To 0?(x=w728) -> (x = 0?=w727:bool)
        n244 = Select(t=u32 16777225, s=w727, f=u32 16777238) -> (s? t:f=w731:u32)
        n245 = property on="Table" class="MCListbox (strict)"("ActiveCell"=w735, "Justify"=enum16{"Left", "Center", "Right"}."Center" ("Active Cell:Cell Justification"), "CellBG"=w731) -> ()  [unwired: 2 in, 2 out]
      }
    }
    frame Enabled {
    }
  }
